vi "presion.vi"(9 "error in (no error)":errorcluster, 10 "COM Bluegiga in":refnum<visa-resource-name>) -> (0 "error out":errorcluster, 1 "Presión":dbl, 3 "COM Bluegiga out":refnum<visa-resource-name>)   [LabVIEW 2020]
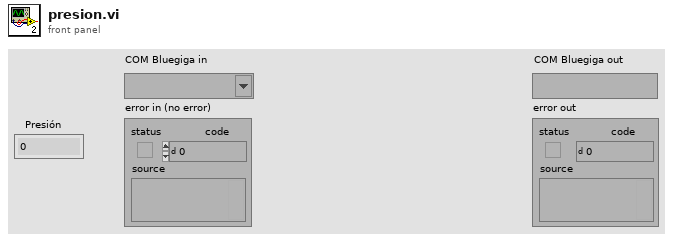
[diagram p1: front panel]
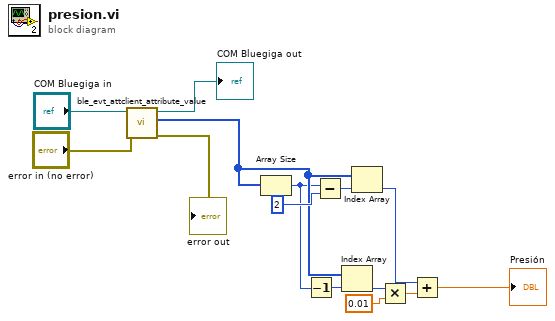
[diagram p0: block diagram]
diagram:
  n1 = call <vilib>:"ble_evt_attclient_attribute_value.vi"("error in (no error)"="error in (no error)", "COM Bluegiga in"="COM Bluegiga in") -> ("error out"=→"error out":errorcluster, "characteristic value"=w12:u8[], "COM Bluegiga out"=→"COM Bluegiga out":refnum<visa-resource-name>)  [unwired: 6 in, 1 out]
  n2 = Array Size(array=w12) -> (size(s)=w10:i32)
  n3 = Decrement(x=w10) -> (x-1=w11:i32)
  n4 = Subtract(x=w10, y=2) -> (x-y=w14:i32)
  n5 = Index Array(array=w12, index=w11) -> (element=w9:u8)
  n6 = Index Array(array=w12, index=w14) -> (element=w6:u8)
  n7 = Multiply(x=w9, y=0.01) -> (x*y=w7:dbl)
  n8 = Add(x=w6, y=w7) -> (x+y=→"Presión":dbl)
